vi "Initialize Oauth for Harvest.vi"(6 "Refresh Token":string, 8 "Account ID":string, 9 "Harvest Access Scope":T1={"all"=TRUE, "harvest:all"=FALSE, "forercast:all"=FALSE, "harvest:{accountID}"=FALSE, "forercast:{accountID}"=FALSE}, 10 "Client Secret":string, 11 "Client ID":string) -> (0 "error out":errorcluster, 3 "Oauth2.Harvest":refnum<class "Oauth2.Harvest.lvclass">)   [LabVIEW 2020, in "Oauth2.Harvest.lvclass"]
uses:
  Oauth2.Harvest.lvclass
  C:/Data/1_Projects/CIGH_Oauth2/source/Oauth2/Oauth2.lvclass
  Oauth2/Oauth2.lvclass
  <vilib>/LabVIEW Open Source Project/Data Manipulation/Variant/OpenVariant.lvlib
  Harvest Access Scopes.ctl
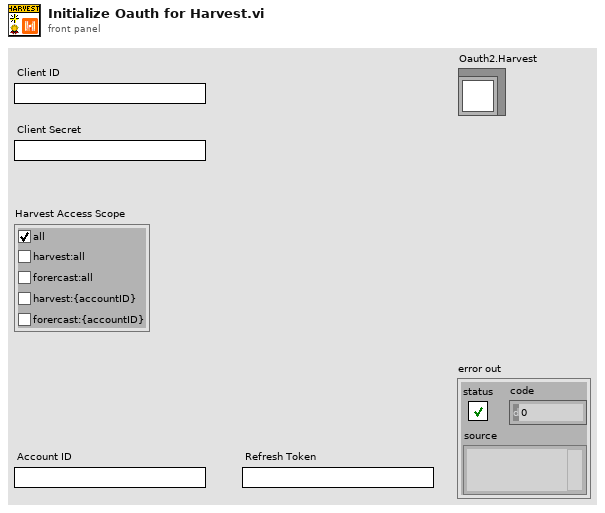
[diagram p1: front panel]
types:
  T1 = typedef "Oauth2.Harvest.lvclass/Harvest Access Scopes.ctl" = cluster{"all":bool, "harvest:all":bool, "forercast:all":bool, "harvest:{accountID}":bool, "forercast:{accountID}":bool}
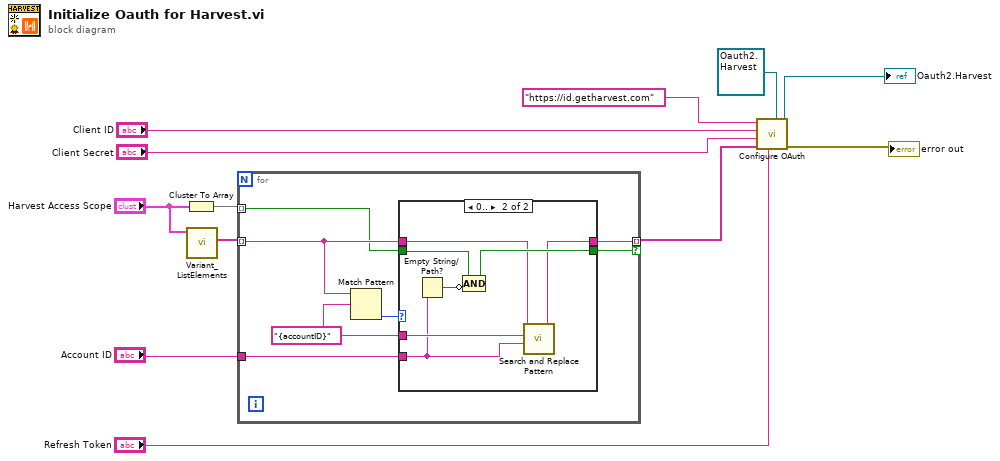
[diagram p0: block diagram]
diagram:
  n1 = Cluster To Array(cluster="Harvest Access Scope") -> (array=w11:bool[])
  n2 = call <vilib>:"Variant_ListElements.vi"("Variant"="Harvest Access Scope") -> ("element names"=w12:string[])  [unwired: 7 in, 3 out]
  n3 = for {
    tunnel: [w17] -> w10 mode=indexing if=w16
    tunnel: w12 -> [w18] mode=indexing
    tunnel: w11 -> [w15] mode=indexing
    tunnel: "Account ID" -> [w14]
    w13 = "{accountID}" ("regular expression")
    n4 = Match Pattern(string=w18, regular expression=w13) -> (offset past match=w19:i32)  [unwired: 1 in, 3 out]
    n5 = case shown="0.." w19 {
      tunnel: w18 -> [w21 w25]
      tunnel: [w21 w24] -> w17
      tunnel: [w20 w26] -> w16
      tunnel: w15 -> [w20 w27]
      tunnel: w14 -> [_ w22]
      tunnel: w13 -> [_ w23]
      frame Default {
      }
      frame 0.. {
        n6 = Empty String/Path?(string/path=w22) -> (empty?=w28:bool)
        n7 = Compound Arithmetic op=AND(w27, invert w28) -> (w26:bool)
        n8 = call-poly <vilib>:"Search and Replace Pattern.vi"("string"=w25, "regular expression (\"\")"=w23, "replace string (\"\")"=w22) -> ("result string"=w24:string)  [unwired: 2 in, 1 out]
      }
    }
  }
  n9 = call "Configure OAuth.vi"("Oauth2 in"=refnum<class "Oauth2.Harvest.lvclass"> refnum ("Oauth2.Harvest in"), "Refresh Token"="Refresh Token", "scopes"=w10, "Client Secret"="Client Secret", "Client ID"="Client ID", "Authorization Server URI"="https://id.getharvest.com" ("path")) -> ("error out"=→"error out":errorcluster, "Oauth2"=→"Oauth2.Harvest":refnum<class "Oauth2.Harvest.lvclass">)  [unwired: 4 in]
